vi "Histogram2DManual0008.vi"   [LabVIEW 2013]
uses:
  ModeType.ctl
  <vilib>/Heliosphere Research LLC/Advanced Plotting Toolkit/api_core/NewPlotScales.ctl
  ErrorCodes.ctl
  <vilib>/Heliosphere Research LLC/Advanced Plotting Toolkit/api_plotting/Histogram2D_Manual.vi
  <vilib>/Heliosphere Research LLC/Advanced Plotting Toolkit/Advanced Plotting Toolkit.lvlib
types:
  T1 = typedef "ErrorCodes.ctl" = u32
  T2 = typedef "Advanced Plotting Toolkit.lvlib/NewPlotScales.ctl" = enum16{"Default", "Linear", "Log", "Symlog"}
  T3 = typedef "ModeType.ctl" = enum16{"Normal", "Expected Failure", "Skipped", "Broken"}
  T4 = typedef "Advanced Plotting Toolkit.lvlib/PlotID.ctl" = i32
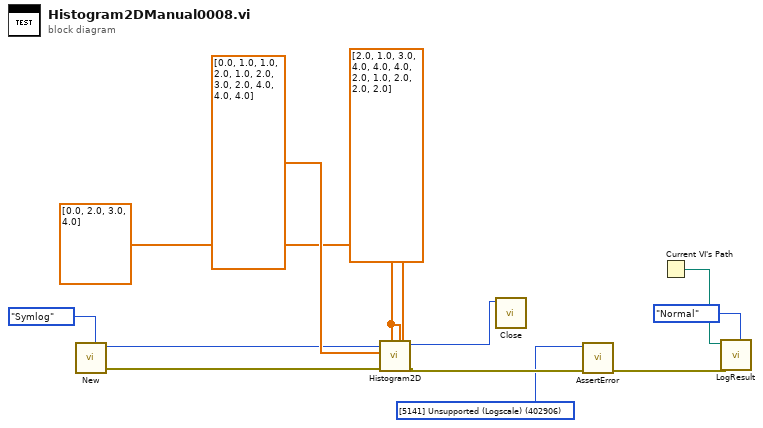
[diagram p0: block diagram]
diagram:
  w1 = T1 402906 items=["[5120] Invalid ID"=402902, "[5110] Failed to Init"=402900, "[5111] Unknown Error"=402901, "[5130] Save - Bad File Extension"=402403, "[5131] Save - General Error"=402904, "[5140] Unsupported (Polar)"=402905, "[5141] Unsupported (Logscale)"=402906, "[5142] Coordinates Not Regular"=402907] ("Expected Error")
  w8 = dbl[] [0.0, 2.0, 3.0, 4.0] ("X Bin Edges")
  n1 = call <vilib>:"New.vi"("Y Axis Scale"=NewPlotScales."Symlog") -> ("error out"=w5:errorcluster, "Plot ID"=w6:T4)  [unwired: 9 in]
  n2 = call-poly <vilib>:"Histogram2D.vi"("Y Bin Edges"=w8, "X Bin Edges"=w8, "error in (no error)"=w5, "Y Data"=dbl[] [2.0, 1.0, 3.0, 4.0, 4.0, 4.0, 2.0, 1.0, 2.0, 2.0, 2.0] ("X Data"), "X Data"=dbl[] [0.0, 1.0, 1.0, 2.0, 1.0, 2.0, 3.0, 2.0, 4.0, 4.0, 4.0], "Plot ID"=w6) -> ("error out"=w4:errorcluster, "Plot ID Out"=w3:T4)  [unwired: 4 in]
  n3 = call <vilib>:"Close.vi"("Plot ID"=w3) -> ()  [unwired: 10 in, 1 out]
  n4 = call "AssertError.vi"("error in (no error)"=w4, "Expected Error"=w1) -> ("error out"=w2:errorcluster)  [unwired: 9 in]
  n5 = Current VI's Path() -> (path=w12:path)
  n6 = call "LogResult.vi"("Mode"=ModeType."Normal", "Test Result"=w2, "VI Path"=w12) -> ()  [unwired: 9 in]
